vi "FlattenLFCoeffs.vi"(8 "FlattenSourceEnd(Hz)":dbl=5.0, 9 "FlattenSourceStart(Hz)":dbl=2.0, 10 "Values":dbl[](array[numeric]), 11 "Frequencies":dbl[](array[numeric])) -> (2 "LF-flattenedValues":dbl[](array[numeric]))   [LabVIEW 2011]
uses:
  <vilib>/Analysis/NI_AALBase.lvlib
panel:
  out "XY Graph":cluster{"Frequencies":dbl[], dbl[]}[](graph)
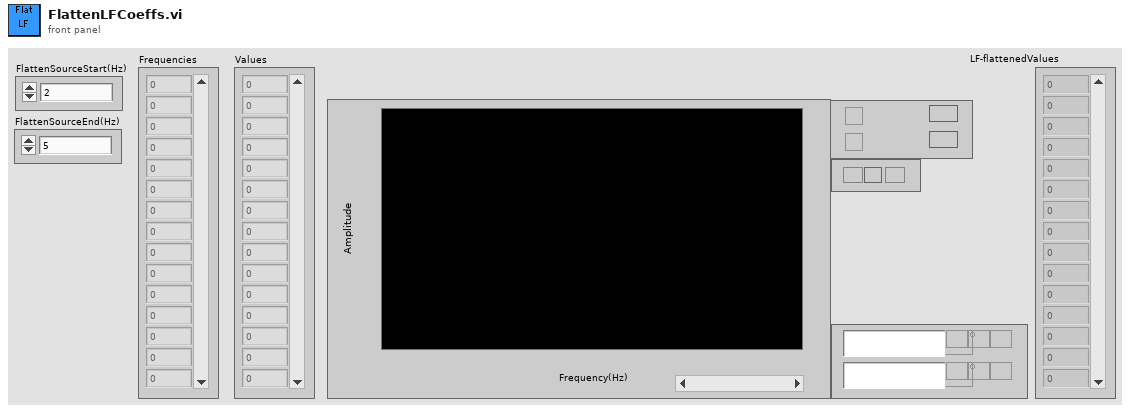
[diagram p1: front panel]
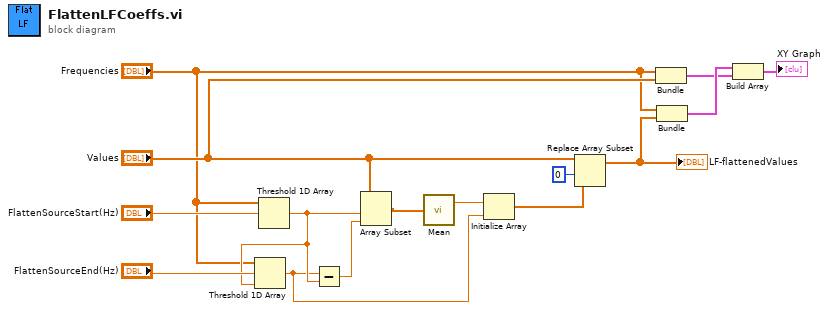
[diagram p0: block diagram]
diagram:
  n1 = Threshold 1D Array(2:"FlattenSourceStart(Hz)", 3:"Frequencies") -> (0:w10:dbl)  [unwired: 1 in]
  n2 = Threshold 1D Array(1:w10, 2:"FlattenSourceEnd(Hz)", 3:"Frequencies") -> (0:w1:dbl)
  n3 = Subtract(x=w1, y=w10) -> (x-y=w5:dbl)
  n4 = Array Subset(array="Values", index=w10, length=w5) -> (w9:dbl[])
  n5 = call <vilib>:"Mean.vi"("X"=w9) -> ("mean"=w6:dbl)  [unwired: 1 out]
  n6 = Initialize Array(w6, w1) -> (w4:dbl[])
  n7 = Replace Array Subset(array="Values", new element=w4, index=0) -> (w3:dbl[])
  "LF-flattenedValues" <- w3
  n8 = Bundle("Frequencies"="Frequencies", "Values"="Values") -> (w13:cluster{"Frequencies":dbl[], "Values":dbl[]})  [unwired: 1 in]
  n9 = Bundle("Frequencies"="Frequencies", "Values"=w3) -> (w14:cluster{"Frequencies":dbl[], "Values":dbl[]})  [unwired: 1 in]
  n10 = Build Array(w14, w13) -> (→"XY Graph":cluster{"Frequencies":dbl[], "Values":dbl[]}[])
